vi "Wait for Request.vi"(8 "error in (no error)":errorcluster, 9 "timeout in ms (100)":i32, 11 "Server in":refnum<class "JSONRPC Server.lvclass">) -> (0 "error out":errorcluster, 1 "timed out?":bool, 2 "Request":refnum<class "Request.lvclass">, 3 "Server out":refnum<class "JSONRPC Server.lvclass">)   [LabVIEW 2015, in "JSONRPC Server.lvclass"]
doc: "This fetches a new request from the client.s"
uses:
  JSONRPC Server.lvclass
  Request/Request.lvclass
  JSONRPC Server.lvclass/JSONRPC Server.ctl
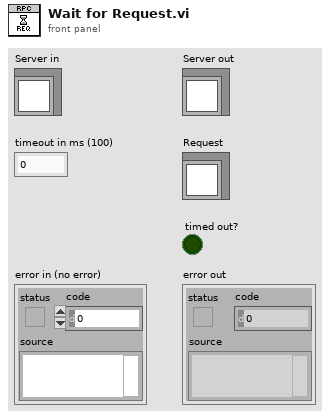
[diagram p1: front panel]
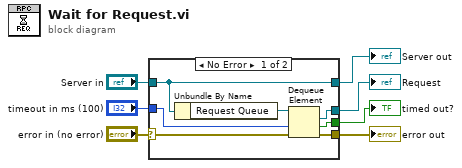
[diagram p0: block diagram]
diagram:
  n1 = case shown="No Error" "error in (no error)" {
    selector: "error in (no error)" -> [w11 w16]
    tunnel: [w9 w16] -> w6
    tunnel: [w14 w15] -> w4
    tunnel: "Server in" -> [w14 w15]
    tunnel: "timeout in ms (100)" -> [w12 _]
    tunnel: [w10 _] -> w2
    tunnel: [w8 _] -> w1
    frame No Error {
      n2 = Unbundle By Name(w14) -> ("Request Queue"=w13:refnum<queue>)
      n3 = Dequeue Element(queue=w13, timeout in ms (-1)=w12, error in (no error)=w11) -> (element=w10:refnum<class "Request.lvclass">, timed out?=w8:bool, error out=w9:errorcluster)  [unwired: 1 out]
    }
    frame Error {
    }
  }
  "error out" <- w6
  "Server out" <- w4
  "Request" <- w2
  "timed out?" <- w1
